vi "BLCDDriving.vi"() -> ()   [LabVIEW 2016]
uses:
  <vilib>/DAQmx/write.llb/DAQmx Write (Digital Bool 1Line 1Point).vi
  <vilib>/DAQmx/write.llb/DAQmx Write (Analog DBL 1Chan 1Samp).vi
  <vilib>/DAQmx/read.llb/DAQmx Read (Analog DBL 1Chan 1Samp).vi
  <vilib>/DAQmx/read.llb/DAQmx Read (Counter DBL 1Chan 1Samp).vi
  <vilib>/DAQmx/miscellaneous.llb/DAQmx Fill In Error Info.vi
panel:
  out "data":dbl format="%0.2f"
  out "error out DIR":errorcluster
  in  "error in DIR":errorcluster
  in  "Right / Left":bool
  out "Druck [bar]":dbl format="%0.2f"
  out "error out 2":errorcluster
  out "error out":errorcluster
  in  "error in":errorcluster
  out "Temperatur [C°]":dbl format="%0.2f"
  in  "error in 2":errorcluster
  out "error out DI":errorcluster
  out "RL":bool
  out "error out RL":errorcluster
  out "error out AO":errorcluster
  in  "AO-Value [V]":dbl(slide) scale=0.0..10.0
  in  "Start / Stop":bool
  in  "error in (no error)":errorcluster
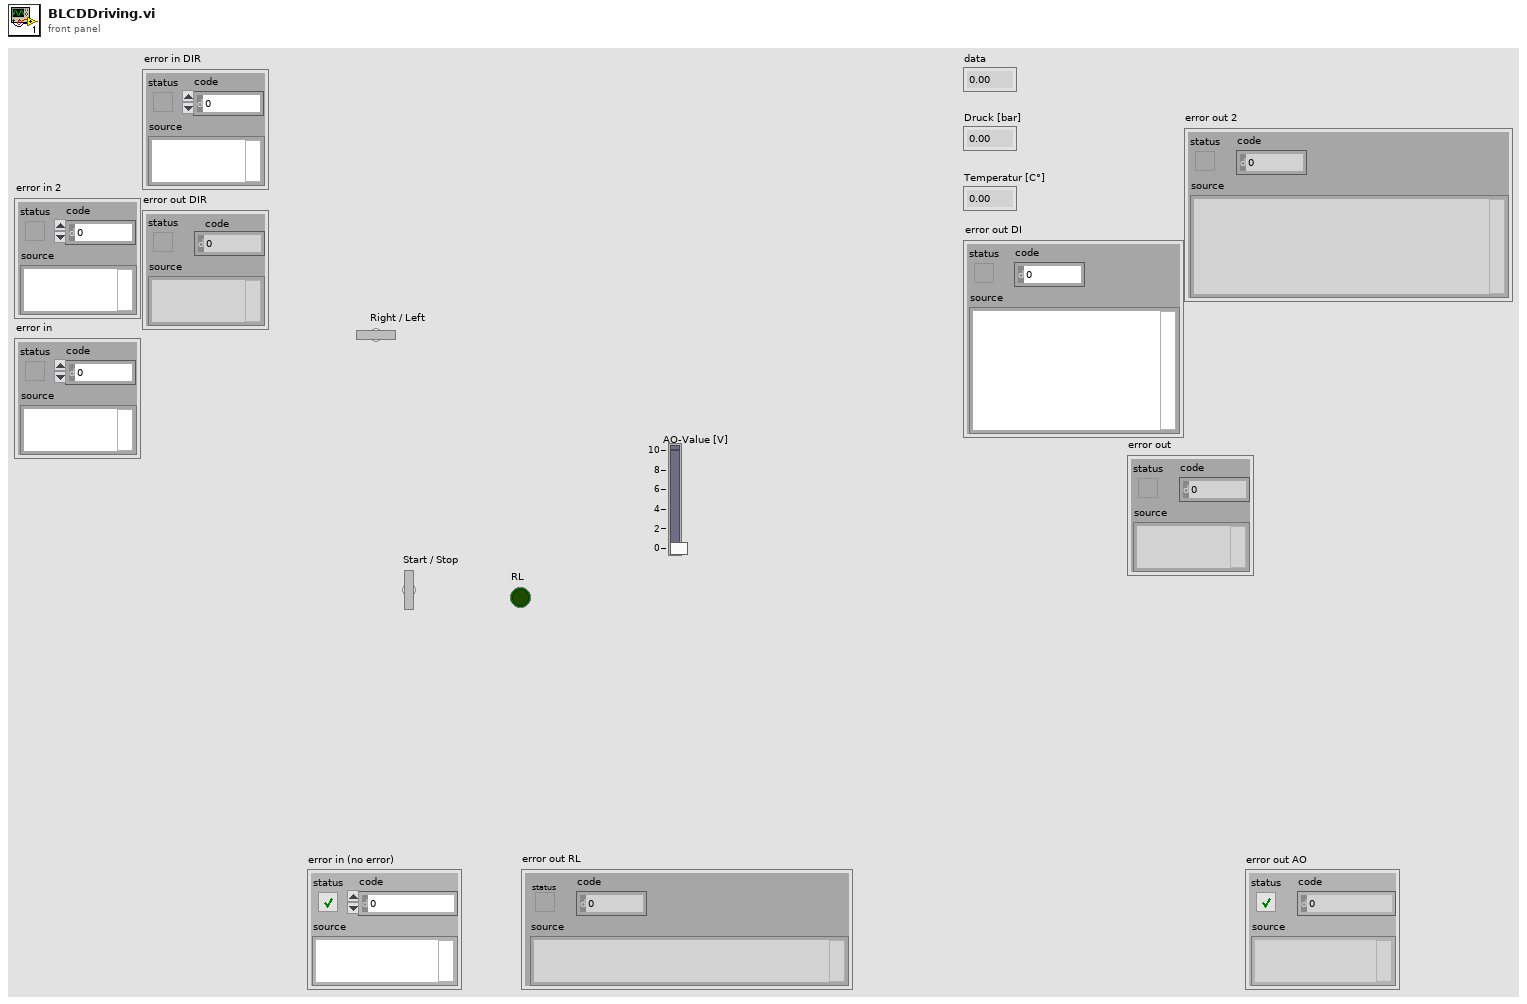
[diagram p1: front panel]
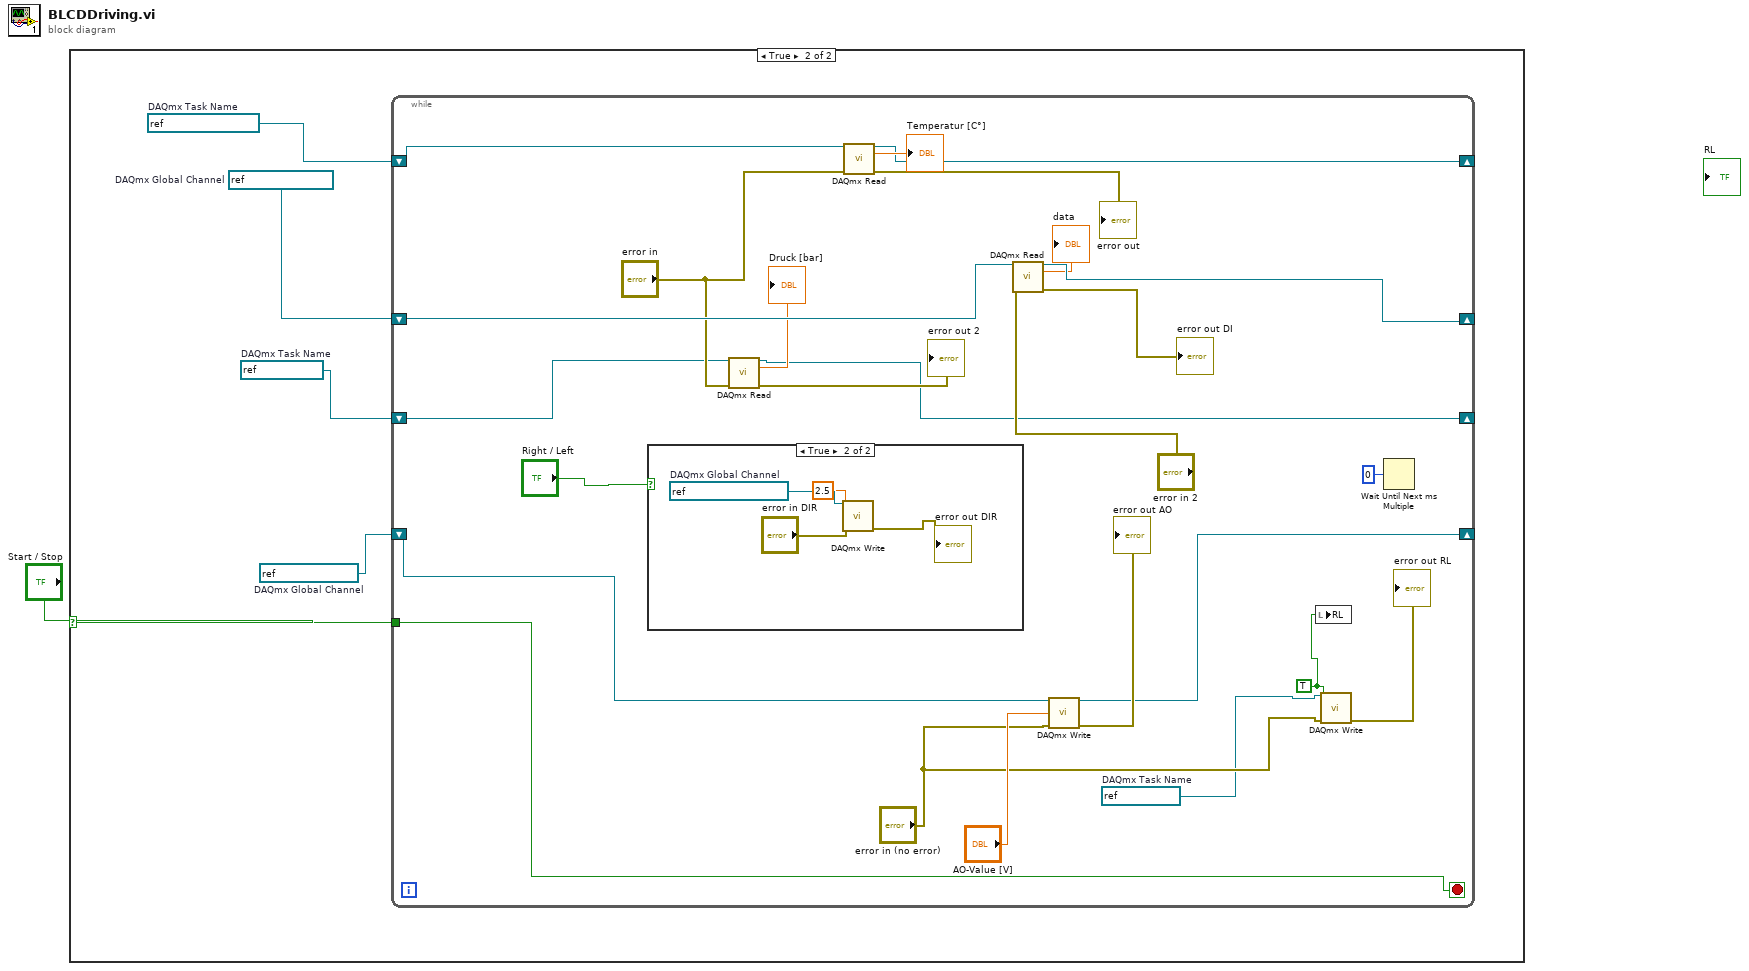
[diagram p0: block diagram]
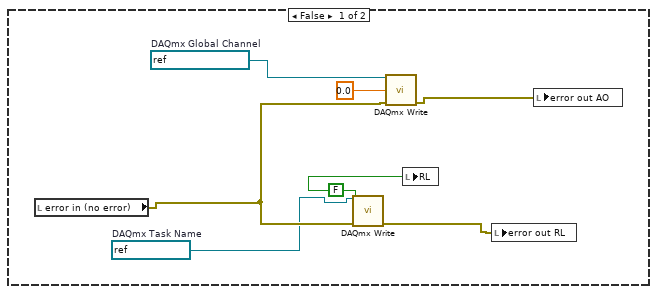
[diagram p2: hidden frame]
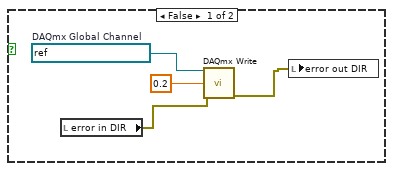
[diagram p3: hidden frame]
diagram:
  n1 = case shown="True" "Start / Stop" {
    selector: "Start / Stop" -> [_ w12]
    frame False {
      w2 = refnum<k21> "RelayTask"  # DAQmx Task Name
      w4 = FALSE ("data")
      w8 = refnum<k21> "SpannungAO"  # DAQmx Global Channel
      n2 = local read "error in (no error)"() -> (w3:errorcluster)
      n3 = call-poly <vilib>:"DAQmx Write.vi"("task/channels in"=w2, "data"=w4, "error in"=w3) -> ("error out"=w5:errorcluster)  [unwired: 10 in, 2 out]
      n4 = call-poly <vilib>:"DAQmx Write.vi"("task/channels in"=w8, "data"=0.0, "error in"=w3) -> ("error out"=w6:errorcluster)  [unwired: 10 in, 2 out]
      n5 = local write "RL"(w4) -> ()
      n6 = local write "error out RL"(w5) -> ()
      n7 = local write "error out AO"(w6) -> ()
    }
    frame True {
      w9 = refnum<k21> "TemperaturTask"  # DAQmx Task Name
      w10 = refnum<k21> "StromTask"  # DAQmx Task Name
      w11 = refnum<k21> "SpannungAO"  # DAQmx Global Channel
      w13 = refnum<k21> "FrequenzKanal"  # DAQmx Global Channel
      n8 = while {
        shift-right: [w29] -> _
        shift-left: w13 -> [w30]
        tunnel: w12 -> [w26]
        shift-right: [w20] -> _
        shift-left: w11 -> [w21]
        shift-right: [w18] -> _
        shift-left: w10 -> [w19]
        shift-right: [w15] -> _
        shift-left: w9 -> [w16]
        shift-right: [w15] -> _
        shift-left: _ -> [_]
        stop <- w26 stop-if-true
        w25 = refnum<k21> "RelayTask"  # DAQmx Task Name
        w33 = TRUE ("data")
        n9 = case shown="True" "Right / Left" {
          frame False {
            w42 = refnum<k21> "SpannungA1_DIR"  # DAQmx Global Channel
            n10 = local read "error in DIR"() -> (w40:errorcluster)
            n11 = call-poly <vilib>:"DAQmx Write.vi"("task/channels in"=w42, "data"=0.2, "error in"=w40) -> ("error out"=w39:errorcluster)  [unwired: 10 in, 2 out]
            n12 = local write "error out DIR"(w39) -> ()
          }
          frame True {
            w46 = refnum<k21> "SpannungA1_DIR"  # DAQmx Global Channel
            n13 = call-poly <vilib>:"DAQmx Write.vi"("task/channels in"=w46, "data"=2.5, "error in"="error in DIR") -> ("error out"=→"error out DIR":errorcluster)  [unwired: 10 in, 2 out]
          }
        }
        n14 = call-poly <vilib>:"DAQmx Read.vi"("task/channels in"=w19, "error in"="error in") -> ("task out"=w18:refnum<k21>, "data"=→"Druck [bar]":dbl, "error out"=→"error out 2":errorcluster)  [unwired: 11 in]
        n15 = call-poly <vilib>:"DAQmx Read.vi"("task/channels in"=w16, "error in"="error in") -> ("task out"=w15:refnum<k21>, "data"=→"Temperatur [C°]":dbl, "error out"=→"error out":errorcluster)  [unwired: 11 in]
        n16 = call-poly <vilib>:"DAQmx Read.vi"("task/channels in"=w30, "error in"="error in 2") -> ("task out"=w29:refnum<k21>, "data"=→"data":dbl, "error out"=→"error out DI":errorcluster)  [unwired: 11 in]
        n17 = call-poly <vilib>:"DAQmx Write.vi"("task/channels in"=w21, "data"="AO-Value [V]", "error in"="error in (no error)") -> ("task out"=w20:refnum<k21>, "error out"=→"error out AO":errorcluster)  [unwired: 10 in, 1 out]
        n18 = local write "RL"(w33) -> ()
        n19 = call-poly <vilib>:"DAQmx Write.vi"("task/channels in"=w25, "data"=w33, "error in"="error in (no error)") -> ("error out"=→"error out RL":errorcluster)  [unwired: 10 in, 2 out]
        n20 = Wait Until Next ms Multiple(millisecond multiple=u32 0) -> ()  [unwired: 1 out]
      }
    }
  }
